vi "Valve 3 position help.vi"(1 "Boolean":bool) -> (0 "Numeric":i32)   [LabVIEW 2017]
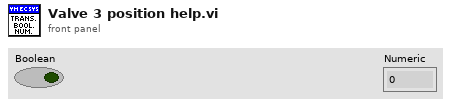
[diagram p1: front panel]
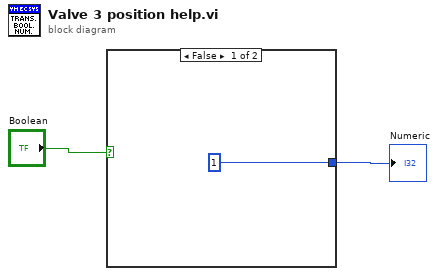
[diagram p0: block diagram]
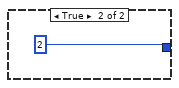
[diagram p2: hidden frame]
diagram:
  n1 = case shown="False" "Boolean" {
    tunnel: [1 2] -> w1
    frame False {
    }
    frame True {
    }
  }
  "Numeric" <- w1
